vi "get advanced system information - example.vi"() -> ()   [LabVIEW 2016, in "SMI.lvlib"]
uses:
  SMI.lvlib
  classes/SysCfg Device/SysCfg Device.lvclass
  classes/Controller/Controller.lvclass
  <resource>/objmgr/nisysapi.rc
  <resource>/objmgr/nicriosae.rc
panel:
  in  "login":cluster{"user name":string, "password":string}={"user name"="admin", "password"=""}
  out "error out":errorcluster
  out "disable RT startup app":bool
  out "system status":string
  out "operating system architecture":string
  in  "IP address (localhost)":string="localhost"
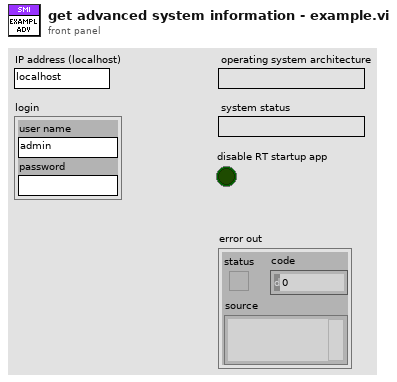
[diagram p1: front panel]
types:
  T1 = typedef "SMI.lvlib/Controller.lvclass/controller information.ctl" = cluster{"system session":refnum<data-value>, "system hardware ref":refnum<data-value>, "vendor name":string, "product name":string, "product ID":u16, "serial number":string, "device information":T2, "primary network adapter":T3, "secondary network adapters":T3[]}
  T2 = typedef "SMI.lvlib/Controller.lvclass/device information.ctl" = cluster{"resource":string, "device class":string, "system start time":timestamp, "current time":timestamp, "time zone":string, "firmware revision":string, "image title":string, "image version":string, "system status":string}
  T3 = typedef "SMI.lvlib/Controller.lvclass/network adapter settings.ctl" = cluster{"IP address":string, "MAC address":string, "IP address request mode":u32, "subnet mask":string, "gateway":string, "DNS server":string, "adapter mode":u32, "adapter type":u32}
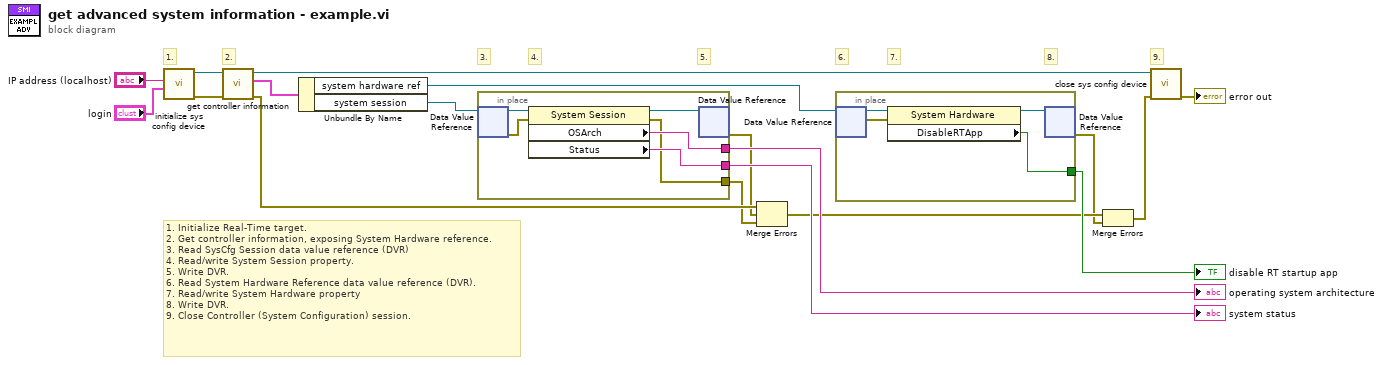
[diagram p0: block diagram]
diagram:
  # "8."
  # "7."
  # "5."
  # "4."
  # "3."
  # "6."
  # "9."
  # "2."
  # "1."
  # "1. Initialize Real-Time target.\n2. Get controller information, exposing System Hardware reference.\n3. Read SysCfg Session data value reference (DVR)\n4. Read/write System Session property.\n5. Write DVR.\n6. Read System Hardware Reference data value reference (DVR).\n7. Read/write System Hardware property\n8. Write DVR.\n9. Close Controller (System Configuration) session."
  n1 = call "initialize sys config device.vi"("login"="login", "IP address (localhost)"="IP address (localhost)") -> ("error out"=w18:errorcluster, "Controller out"=w17:refnum<class "Controller.lvclass">)  [unwired: 8 in]
  n2 = call "get controller information.vi"("error in"=w18, "Controller in"=w17) -> ("error out"=w16:errorcluster, "controller information"=w10:T1, "Controller out"=w4:refnum<class "Controller.lvclass">)  [unwired: 7 in]
  n3 = Unbundle By Name(w10) -> ("system hardware ref"=w6:refnum<data-value>, "system session"=w9:refnum<data-value>)
  n4 = in-place {
    in-place-border: [w21] -> w13
    in-place-border: [w20] -> w14
    in-place-border: [w19] -> w7
    n5 = in-place-dvr #1(w9) -> (w24:refnum<k21>, w22:errorcluster)
    n6 = property class="System Session"(reference=w24, error in=w22) -> (reference out=w23:refnum<k21>, error out=w19:errorcluster, "OSArch"=w20:string, "Status"=w21:string)
    n7 = in-place-dvr #1(w23) -> (w8:errorcluster)  [unwired: 1 out]
  }
  "operating system architecture" <- w14
  "system status" <- w13
  n8 = Merge Errors(w16, w8, w7) -> (w3:errorcluster)
  n9 = in-place {
    in-place-border: [w25] -> w5
    n10 = in-place-dvr #2(w6) -> (w28:refnum<k20>, w27:errorcluster)
    n11 = property class="System Hardware"(reference=w28, error in=w27) -> (reference out=w26:refnum<k20>, "DisableRTApp"=w25:bool)  [unwired: 1 out]
    n12 = in-place-dvr #2(w26) -> (w2:errorcluster)  [unwired: 1 out]
  }
  "disable RT startup app" <- w5
  n13 = Merge Errors(w3, w2) -> (w1:errorcluster)
  n14 = call "close sys config device.vi"("error in"=w1, "Controller in"=w4) -> ("error out"=→"error out":errorcluster)  [unwired: 9 in]
